vi "Build Light Data.vi"(9 "Light State Info":string[](array[string]), 10 "Light Name":string) -> (2 "Light Data":T1)   [LabVIEW 2020, in "LMH-Hue.lvlib"]
uses:
  LMH-Hue.lvlib
  Type Defs/Light Data.ctl
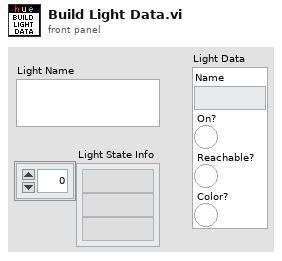
[diagram p1: front panel]
types:
  T1 = typedef "LMH-Hue.lvlib/Light Data.ctl" = cluster{"Name":string, "On?":bool, "Reachable?":bool, "Color?":bool}
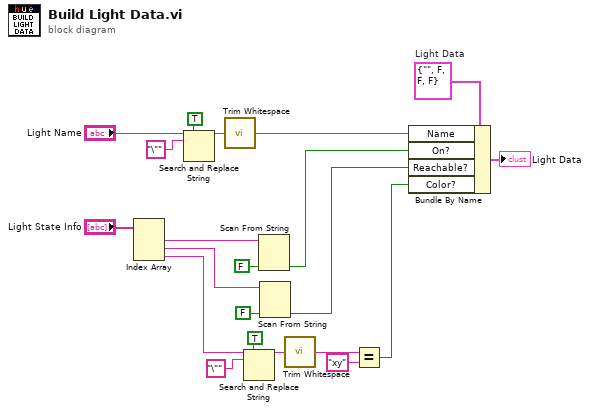
[diagram p0: block diagram]
diagram:
  w21 = T1 {"Name"="", "On?"=FALSE, "Reachable?"=FALSE, "Color?"=FALSE}  # Light Data
  n1 = Index Array(array="Light State Info") -> (element #1=w8:string, element #2=w11:string, element #3=w15:string)  [unwired: 3 in]
  n2 = Search and Replace String(replace all?=TRUE ("replace all? (F)"), input string="Light Name", search string="\"") -> (result string=w5:string)  [unwired: 5 in, 3 out]
  n3 = call <vilib>:"Trim Whitespace.vi"("string"=w5) -> ("trimmed string"=w2:string)  [unwired: 1 in]
  n4 = Search and Replace String(replace all?=TRUE ("replace all? (F)"), input string=w15, search string="\"") -> (result string=w13:string)  [unwired: 5 in, 3 out]
  n5 = Scan From String(input string=w8, default 1=FALSE) -> (output 1=w18:bool)  [unwired: 3 in, 3 out]
  n6 = Scan From String(input string=w11, default 1=FALSE) -> (output 1=w20:bool)  [unwired: 3 in, 3 out]
  n7 = call <vilib>:"Trim Whitespace.vi"("string"=w13) -> ("trimmed string"=w17:string)  [unwired: 1 in]
  n8 = Equal?(x=w17, y="xy") -> (x = y?=w19:bool)
  n9 = Bundle By Name(cluster=w21, "Name"=w2, "On?"=w18, "Reachable?"=w20, "Color?"=w19) -> (→"Light Data":T1)
